vi "Add BOM Tree Row.vi"(8 "error in (no error)":errorcluster, 9 "Parent Tag":string, 10 "BOM Table Raw Items":T1, 11 "TreeControl in":refnum<vi>) -> (0 "error out":errorcluster, 2 "New Item Tag":string, 3 "TreeControl out":refnum<vi>)   [LabVIEW 2018]
uses:
  TypeDef/BOM Table Raw Items.ctl
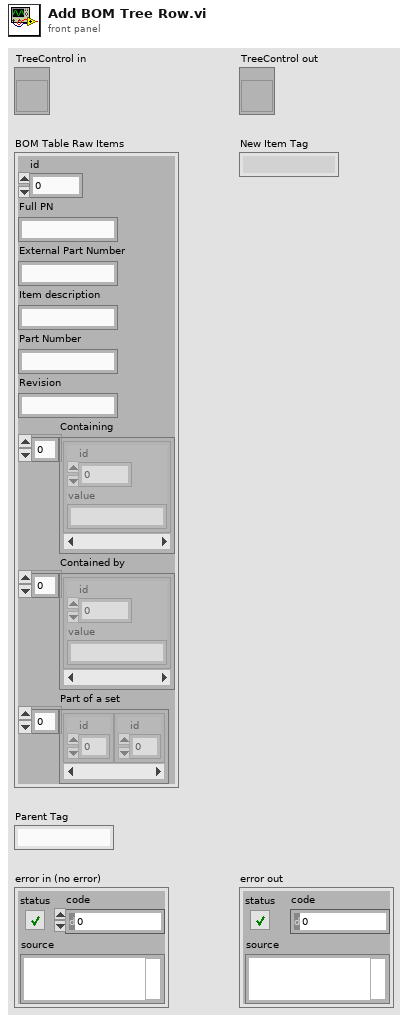
[diagram p1: front panel]
types:
  T1 = typedef "BOM Table Raw Items.ctl" = cluster{"id":i32, "Full PN":string, "External Part Number":string, "Item description":string, "Part Number":string, "Revision":string, "Containing":cluster{"id":i32, "value":string}[], "Contained by":cluster{"id":i32, "value":string}[], "Part of a set":cluster{"id":i32}[]}
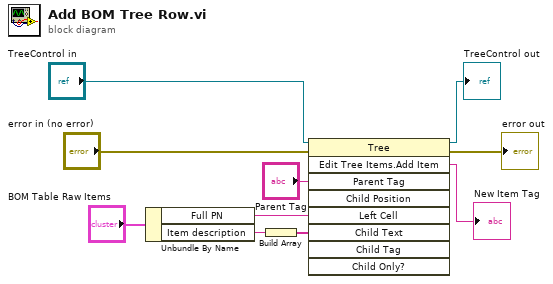
[diagram p0: block diagram]
diagram:
  n1 = Unbundle By Name("BOM Table Raw Items") -> ("Full PN"=w3:string, "Item description"=w4:string)
  n2 = Build Array(w4) -> (w5:string[])
  n3 = invoke class="Tree" method="Edit Tree Items.Add Item"(reference="TreeControl in", error in="error in (no error)", "Parent Tag"="Parent Tag", "Left Cell"=w3, "Child Text"=w5) -> (reference out=→"TreeControl out":refnum<vi>, error out=→"error out":errorcluster, "Edit Tree Items:Add Item"=→"New Item Tag":string)  [unwired: 4 in, 6 out]
